vi "Database Sending.vi"(11 "Command":string) -> ()   [LabVIEW 2024]
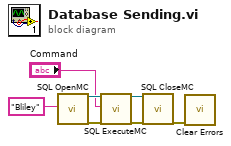
[diagram p0: block diagram]
diagram:
  n1 = call "SQL OpenMC.vi"("ConnectionString In"="Bliley") -> ("Connection Out"=w7:refnum<k7>, "Error out"=w6:errorcluster)  [unwired: 17 in]
  n2 = call "SQL ExecuteMC.vi"("Connection In"=w7, "SQL Query"="Command", "Error in (no error)"=w6) -> ("Connection Out"=w5:refnum<k7>, "Error out"=w4:errorcluster)  [unwired: 15 in]
  n3 = call "SQL CloseMC.vi"("Connection In"=w5, "Error in (no error)"=w4) -> ("Error out"=w2:errorcluster)  [unwired: 17 in]
  n4 = call <vilib>:"Clear Errors.vi"("error in (no error)"=w2) -> ()  [unwired: 5 in, 2 out]
